vi "Report Stop.vi"(8 "error in (no error)":errorcluster, 11 "Module in":refnum<class "Module.lvclass">) -> (0 "error out":errorcluster, 3 "Module out":refnum<class "Module.lvclass">)   [LabVIEW 2020, in "Volatus.lvlib" / "Module.lvclass"]
uses:
  Module.lvclass
  Module.lvclass/Module.ctl
  Event Level.ctl
  Volatus.lvlib
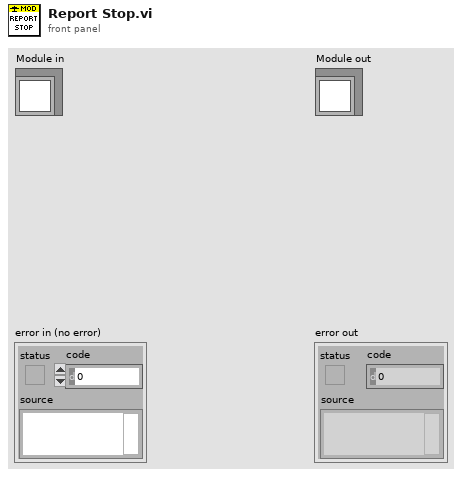
[diagram p1: front panel]
types:
  T1 = typedef "Volatus.lvlib/Event Level.ctl" = enum16{"Debug", "Info", "Warning", "Error"}
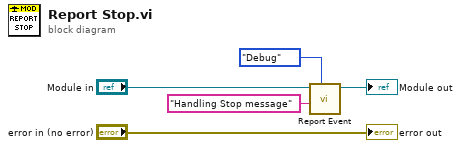
[diagram p0: block diagram]
diagram:
  n1 = call "Report Event.vi"("Level (Info)"=Event_Level."Debug", "Message"="Handling Stop message", "Module in"="Module in") -> ("Module out"=→"Module out":refnum<class "Module.lvclass">)  [unwired: 7 in, 1 out]
  "error out" <- "error in (no error)"
